vi "user initialization.vi"(8 "error in":errorcluster, 10 "configuration in":refnum<class "control module configuration.lvclass">, 11 "fixed channel runtime in":refnum<class "AppStateMachine runtime.lvclass">) -> (0 "error out":errorcluster, 3 "fixed channel runtime out":refnum<class "AppStateMachine runtime.lvclass">)   [LabVIEW 2017, in "AppStateMachine runtime.lvclass"]
uses:
  AppStateMachine runtime.lvclass
  <vilib>/NI/DCAF/Tag Editor Core/control module/configuration/control module configuration.lvclass
  <vilib>/NI/DCAF/addons/InstructionFrameworkSupport/FPGA_FGV_action.ctl
  <vilib>/userdefined/High Color/nirio_resource_hc.ctl
  StateId.ctl
  State.ctl
  LED_Color.ctl
  FPGA/FPGAtypedef.ctl
  configuration/AppStateMachine configuration.lvclass
  C:/Program Files (x86)/National Instruments/LabVIEW 2017/vi.lib/NI/DCAF/Tag Editor Core/control module/configuration/control module configuration.lvclass
  configuration/AppStateMachine configuration.lvclass/AppStateMachine configuration.ctl
  AppStateMachine runtime.lvclass/AppStateMachine runtime.ctl
  configuration/Read PrechargeTimeout.vi
  configuration/Read SynchronizeTimeout.vi
  configuration/Read DCLinkSteadyStateTimeout.vi
  configuration/Read PrechargeLevel.vi
  configuration/Read DCLinkSteadyState.vi
  <instrlib>/_niInstr/FIFO Register Bus/v1/Host/niInstr FIFO Register Bus v1 Host.lvclass
  C:/Program Files (x86)/National Instruments/LabVIEW 2017/instr.lib/_niInstr/Instruction Framework/v1/Host/Instruction Target/niInstr Instruction Target v1 Host.lvclass
  <vilib>/Utility/error.llb/Error Cluster From Error Code.vi
  <vilib>/rvi/errors/niLvFpgaAdjustHostInterfaceError.vi
  <vilib>/rvi/interface/nirviReadWriteControl/nirviReadWriteControl.xnode
  <vilib>/NI/DCAF/Tag Editor Core/control module/runtime/control module runtime.lvclass
  <vilib>/NI/NI JSONRPC Server Framework/Classes/Server/JSONRPC Server.lvclass
  <vilib>/NI/PowerElectronicsControl/ThreePhasePLL/Interface/ThreePhasePLLInterface.lvlib
  <vilib>/NI/PowerElectronicsControl/ActiveFrontEnd/AFE_Interface/AFE_interface.lvlib
  <vilib>/NI/PowerElectronicsControl/Buck-Boost/RealTime/BuckBoostInterface.lvlib
  NiFpgaLv.dll
  <vilib>/rvi/interface/Simulation/niFpgaSimulationCallBeginRW.vi
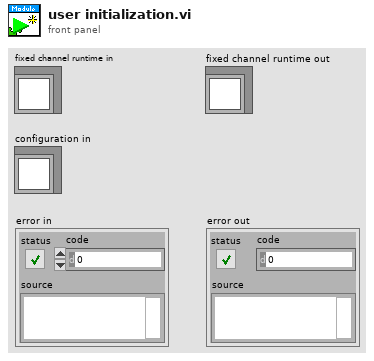
[diagram p1: front panel]
types:
  T1 = typedef "AppStateMachine runtime.lvclass/FPGAtypedef.ctl" = refnum<k20>
  T2 = typedef "AppStateMachine runtime.lvclass/State.ctl" = cluster{"StateId":T3, "LED_Enable":bool, "LED_BlinksPerCycle":i32, "LED_Color":T4, "ResourceUsage":cluster{"CPU":dbl, "Memory":dbl, "Disk":dbl}, "locked":bool, "Detected Frequency":dbl, "VDCLink":dbl, "VLoad":dbl, "Fault Registers":u64, "afeEnabled":bool, "buckboostEnabled":bool, "timer":u32, "PrechargeTimeout":u32, "SynchronizeTimeout":u32, "DCLinkSteadyState":dbl, "PrechargeLevel":dbl, "DCLinkSteadyStateTimeout":u32, "ILoad":dbl}
  T3 = typedef "AppStateMachine runtime.lvclass/StateId.ctl" = enum16{"Initialize", "Idle", "TunePLL", "TuneAFE", "TuneBuckBoost", "Precharge", "Synchronize", "Ready", "EnableAFE", "EnableBuckBoost", "Powered", "SafeState", "UnrecoverableSafeState"}
  T4 = typedef "AppStateMachine runtime.lvclass/LED_Color.ctl" = enum16{"Green", "Yellow"}
  T5 = typedef "nirio_resource_hc.ctl" = tag
  T6 = typedef "FPGA_FGV_action.ctl" = enum16{"get FPGA", "set FPGA", "Close"}
  T7 = typedef "ThreePhasePLLInterface.lvlib/InterfaceRef.ctl" = cluster{"instruction target":refnum<class "niInstr Instruction Target v1 Host.lvclass">, "context":refnum<class "niInstr Instruction Framework Context v1 Host.lvclass">}
  T8 = typedef "AFE_interface.lvlib/InterfaceRef.ctl" = cluster{"instruction target":refnum<class "niInstr Instruction Target v1 Host.lvclass">, "context":refnum<class "niInstr Instruction Framework Context v1 Host.lvclass">}
  T9 = typedef "BuckBoostInterface.lvlib/Interface.ctl" = cluster{"instruction target":refnum<class "niInstr Instruction Target v1 Host.lvclass">, "BuckBoostContext":refnum<class "niInstr Instruction Framework Context v1 Host.lvclass">}
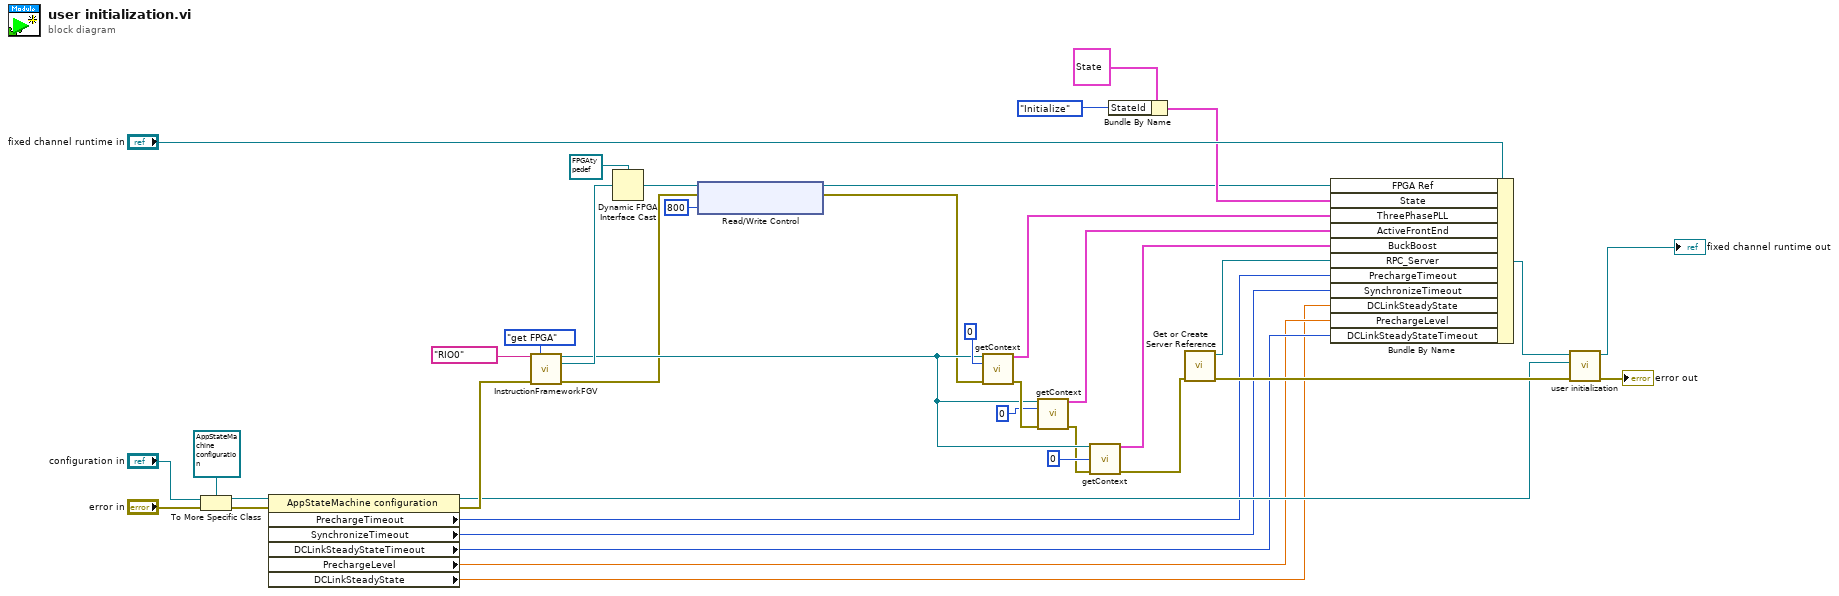
[diagram p0: block diagram]
diagram:
  n1 = To More Specific Class(target class=refnum<class "AppStateMachine configuration.lvclass"> refnum ("AppStateMachine configuration"), reference="configuration in", error in="error in") -> (specific class reference=w13:refnum<class "AppStateMachine configuration.lvclass">, error out=w14:errorcluster)
  n2 = property class="AppStateMachine configuration"(reference=w13, error in=w14) -> (reference out=w11:refnum<class "AppStateMachine configuration.lvclass">, error out=w12:errorcluster, "PrechargeTimeout"=w10:u32, "SynchronizeTimeout"=w9:u32, "DCLinkSteadyStateTimeout"=w8:u32, "PrechargeLevel"=w7:dbl, "DCLinkSteadyState"=w6:dbl)
  n3 = call <vilib>:"InstructionFrameworkFGV.vi"("RIO resource"=T5 "RIO0", "Action"=FPGA_FGV_action."get FPGA", "error in"=w12) -> ("session out"=w26:refnum<class "niInstr FIFO Register Bus v1 Host.lvclass">, "bitfile"=w32:refnum<k20>, "error out"=w4:errorcluster)  [unwired: 10 in]
  n4 = Dynamic FPGA Interface Cast(Session In=T1 refnum ("FPGA typedef"), Type=w32) -> (Session Out=w5:T1)
  n5 = xnode "Read/Write Control"("FPGA VI Reference In"=w5, "error in"=w4, "desiredBuckBoostRate"=u32 800) -> ("FPGA VI Reference Out"=w2:T1, "error out"=w1:errorcluster)
  n6 = call <vilib>:"getContext.vi"("instruction target in"=w26, "instance"=u8 0, "error in"=w1) -> ("Interface"=w33:T7, "error out"=w30:errorcluster)  [unwired: 11 in]
  n7 = call <vilib>:"getContext.vi"("instruction target in"=w26, "instance"=u8 0, "error in"=w30) -> ("Interface"=w28:T8, "error out"=w24:errorcluster)  [unwired: 11 in]
  n8 = call <vilib>:"getContext.vi"("instruction target in"=w26, "instance"=u8 0, "error in"=w24) -> ("Interface"=w22:T9, "error out"=w23:errorcluster)  [unwired: 11 in]
  n9 = Bundle By Name(cluster=T2 {"StateId"=enum."Initialize", "LED_Enable"=FALSE, "LED_BlinksPerCycle"=0, "LED_Color"=enum."Green", "ResourceUsage"={"CPU"=0.0, "Memory"=0.0, "Disk"=0.0}, "locked"=FALSE, "Detected Frequency"=0.0, "VDCLink"=0.0, "VLoad"=0.0, "Fault Registers"=0, "afeEnabled"=FALSE, "buckboostEnabled"=FALSE, "timer"=0, "PrechargeTimeout"=0, "SynchronizeTimeout"=0, "DCLinkSteadyState"=0.0, "PrechargeLevel"=0.0, "DCLinkSteadyStateTimeout"=0, "ILoad"=0.0} ("State"), "StateId"=StateId."Initialize" ("State")) -> (w35:T2)
  n10 = call <vilib>:"Get or Create Server Reference.vi"("error in (no error)"=w23) -> ("error out"=w20:errorcluster, "Server Out"=w27:refnum<class "JSONRPC Server.lvclass">)  [unwired: 9 in]
  n11 = Bundle By Name(cluster="fixed channel runtime in", "FPGA Ref"=w2, "State"=w35, "ThreePhasePLL"=w33, "ActiveFrontEnd"=w28, "BuckBoost"=w22, "RPC_Server"=w27, "PrechargeTimeout"=w10, "SynchronizeTimeout"=w9, "DCLinkSteadyState"=w6, "PrechargeLevel"=w7, "DCLinkSteadyStateTimeout"=w8) -> (w19:refnum<class "AppStateMachine runtime.lvclass">)
  n12 = call-parent "user initialization.vi"("error in"=w20, "configuration in"=w11, "fixed channel runtime in"=w19) -> ("error out"=→"error out":errorcluster, "fixed channel runtime out"=→"fixed channel runtime out":refnum<class "AppStateMachine runtime.lvclass">)  [unwired: 7 in]
